vi "createDataPointScript.vi"(8 "error in (no error)":errorcluster, 10 "script_comment":string) -> (0 "error out":errorcluster, 3 "DataPointScript out":refnum<class "DataPointScript.lvclass">)   [LabVIEW 2009, in "Tools.lvlib" / "Scripting.lvlib" / "DataPointScript.lvclass"]
uses:
  DataPointScript.lvclass
  DataPointScript.lvclass/DataPointScript.ctl
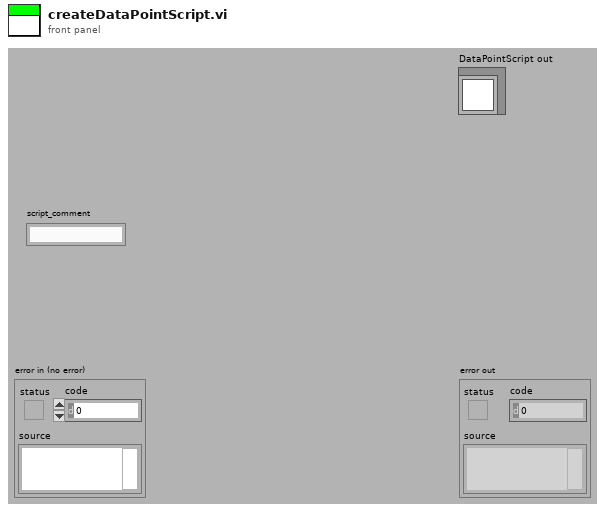
[diagram p1: front panel]
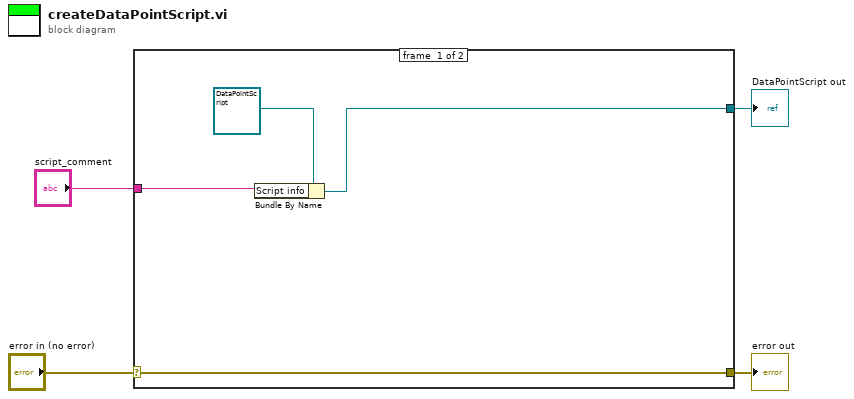
[diagram p0: block diagram]
diagram:
  n1 = case shown="No Error" "error in (no error)" {
    selector: "error in (no error)" -> [w8 w9]
    tunnel: [w8 w9] -> w3
    tunnel: [w5 _] -> w2
    tunnel: "script_comment" -> [w7 _]
    frame #0 {
      n2 = Bundle By Name(cluster=refnum<class "DataPointScript.lvclass"> refnum ("Tools.lvlib:Scripting.lvlib:DataPointScript.lvclass"), "Script info"=w7) -> (w5:refnum<class "DataPointScript.lvclass">)
    }
    frame #1 {
    }
  }
  "error out" <- w3
  "DataPointScript out" <- w2
